vi "START_STOP_2_FILE.vi"(10 "Template":path, 11 "MAP":path) -> (3 "Image":T1(plugin-control))   [LabVIEW 2015]
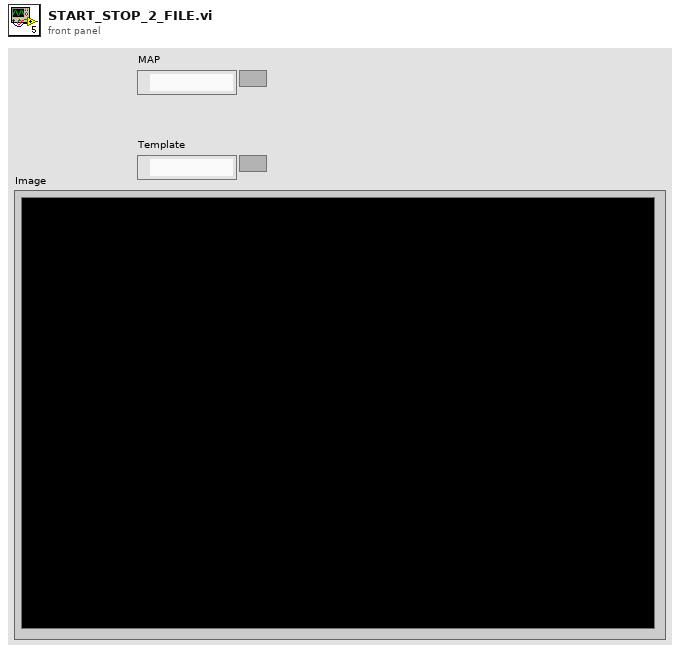
[diagram p1: front panel]
types:
  T1 = typedef "IMAQ Image.ctl" = refnum<image>
  T2 = enum16{"open", "replace", "create", "open or create", "replace or create", "replace or create with confirmation"}
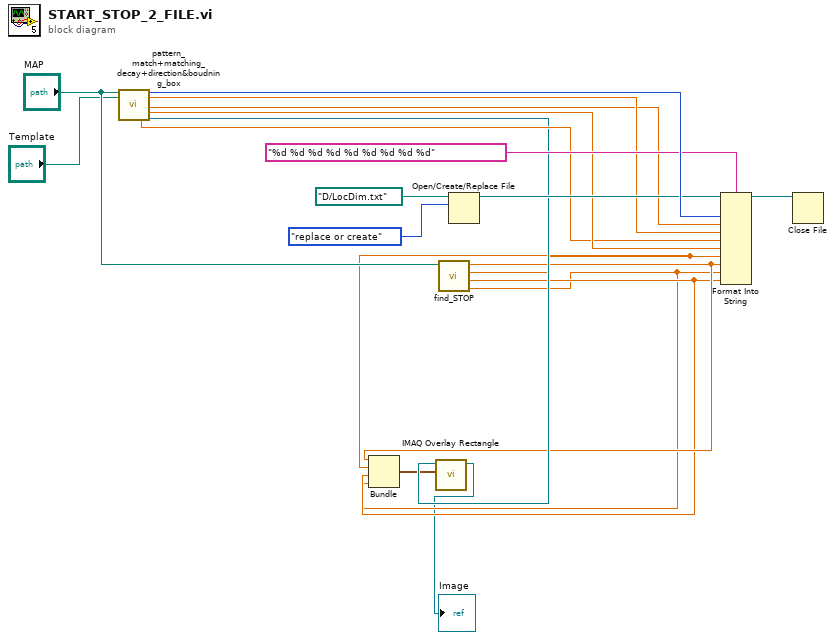
[diagram p0: block diagram]
diagram:
  n1 = call "pattern_match+matching_decay+direction&boudning_box.vi"("Imaginea"="MAP", "Template"="Template") -> ("y 2"=w10:sgl, "Directia"=w17:i32, "x"=w8:sgl, "y"=w7:sgl, "x 2"=w11:sgl, "Image"=w9:T1)  [unwired: 12 in]
  n2 = call "find_STOP.vi"("Path"="MAP") -> ("Y 2"=w3:sgl, "X 2"=w4:sgl, "Y"=w5:sgl, "X"=w6:sgl)  [unwired: 7 in]
  n3 = Bundle("X"=w6, "Y"=w5, "X 2"=w4, "Y 2"=w3) -> (w2:cluster{"X":sgl, "Y":sgl, "X 2":sgl, "Y 2":sgl})  [unwired: 1 in]
  n4 = call "IMAQ Overlay Rectangle"("Rectangle"=w2, "Image"=w9) -> ("Image Out"=→"Image":T1)  [unwired: 8 in, 1 out]
  n5 = Open/Create/Replace File(file path (use dialog)=path "D:/LocDim.txt", operation (0:open)=T2."replace or create") -> (refnum out=w14:refnum<file>)  [unwired: 4 in, 2 out]
  n6 = Format Into String(format string="%d %d %d %d %d %d %d %d %d", initial string=w14, w17, w7, w8, w10, w11, w5, w6, w3, w4) -> (resulting string=w12:refnum<file>)  [unwired: 1 in, 1 out]
  n7 = Close File(refnum=w12) -> ()  [unwired: 1 in, 2 out]
